vi "myRIO_BRig_FPGA_v3,81.vi"() -> ()   [LabVIEW 2014]
uses:
  <vilib>/rvi/Emulation/niFpgaGetClockAttributes.vi
  <vilib>/rvi/Emulation/niFpgaSctlEmulationGetInTimedLoop.vi
  <vilib>/rvi/Emulation/niFpgaEmulationReportErrorSimple.vi
  <vilib>/rvi/eio/common/nirviEmuTemplateMethod_errors.vi
  <vilib>/rvi/Emulation/niFpgaCriticalErrorInLSC.vi
  <vilib>/eio/EIONode/EIONode.xnode
panel:
  in  "L1Led_Baseline":bool
  in  "L2Led_Baseline":bool
  in  "CueLed_Baseline":bool
  in  "I_allReward":bool
  in  "AnaOut_1":u16
  in  "CueLed_Event":bool
  in  "CueLed_nValley":u32=100
  in  "CueLed_nPeak":u32=100
  in  "LC_Event_l2":bool
  in  "LC_Laser_l2":bool
  in  "LC_nShutter_l2":u32=100
  in  "LC_nValley_l2":u32=100
  in  "LC_nPeak_l2":u32=100
  in  "LR_wrong_nDelay_l2":u32
  in  "LR_reward_nDelay_l2":u32
  in  "LR_wrong_nTotal_l2":u32=100
  in  "LR_reward_nTotal_l2":u32=100
  in  "LR_wrong_laser_l2":bool
  in  "LR_wrong_Event_l2":bool
  in  "LR_reward_Laser_l2":bool
  in  "LR_reward_Event_l2":bool
  out "AnaIn_1":u16
  out "AnaIn_0":u16
  out "timeTrial_count":u32
  in  "timeTrial_trig":bool
  in  "k1__counter_per_ms":u16=100 min=100 max=40000 step=1
  in  "LC_nShutter_l1":u32=100
  in  "AnaOut_0":u16
  in  "LC_nValley_l1":u32=100
  in  "LC_nPeak_l1":u32=100
  in  "LC_Event_l1":bool
  in  "LR_wrong_nTotal_l1":u32=100
  in  "LR_wrong_nDelay_l1":u32
  in  "LR_reward_nTotal_l1":u32=100
  in  "LR_reward_nDelay_l1":u32
  in  "LR_reward_Event_l1":bool
  in  "LR_wrong_Event_l1":bool
  out "SelectWrong":bool
  out "SelectReward":bool
  in  "LR_wrong_Laser_l1":bool
  in  "LR_reward_Laser_l1":bool
  in  "Left(F)_or_Right(T)":bool
  in  "ignoreWrong":bool
  in  "SelectionState":bool
  in  "LC_Laser_l1":bool
  in  "FPGA_Stop":bool
  in  "audioTrigger_L":bool
  in  "audioTrigger_R":bool
  in  "audioFreq_L_kHz":u8=14 min=1 max=14 step=1
  in  "audioAmp_L":u16=1 min=1 max=32767 step=1
  in  "audioFreq_R_kHz":u8=14 min=1 max=14 step=1
  in  "audioAmp_R":u16=1 min=1 max=32767 step=1
  in  "A3_SL":bool
  in  "A1_SR":bool
  in  "Counts_Reset":bool
  out "A4_LickR":u32
  out "A2_LickL":u32
  in  "A6_Act":bool
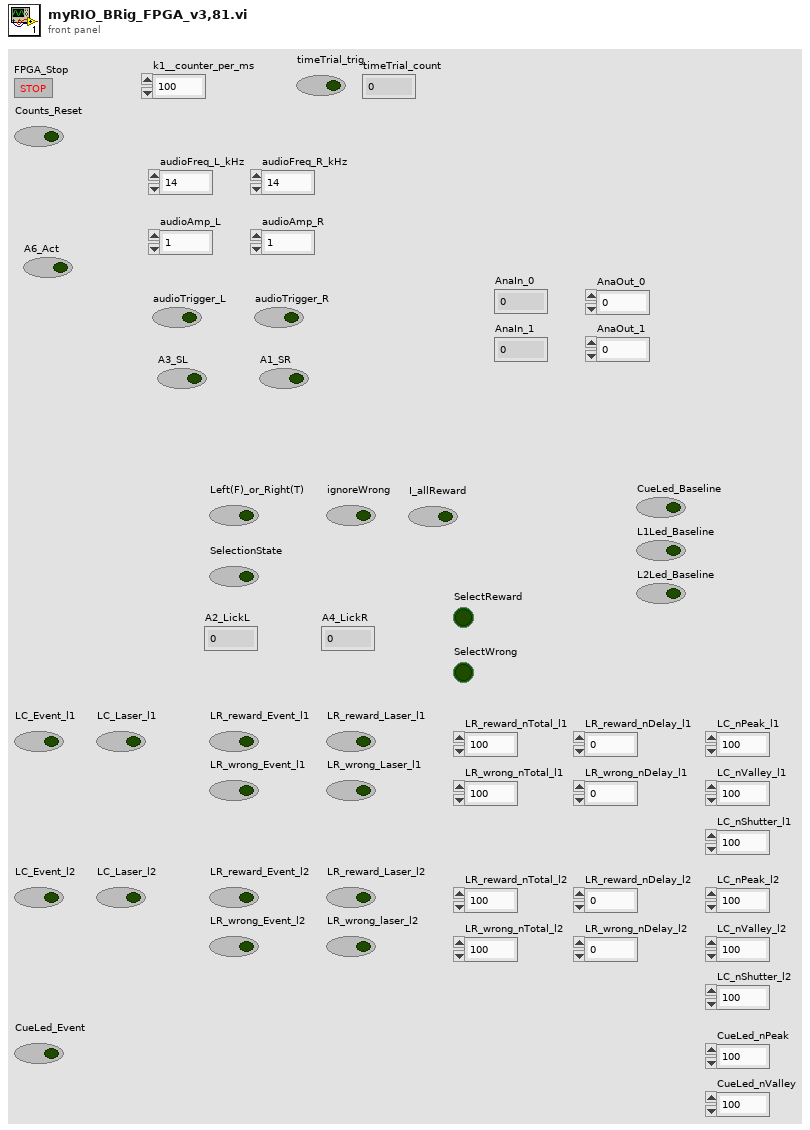
[diagram p1: front panel]
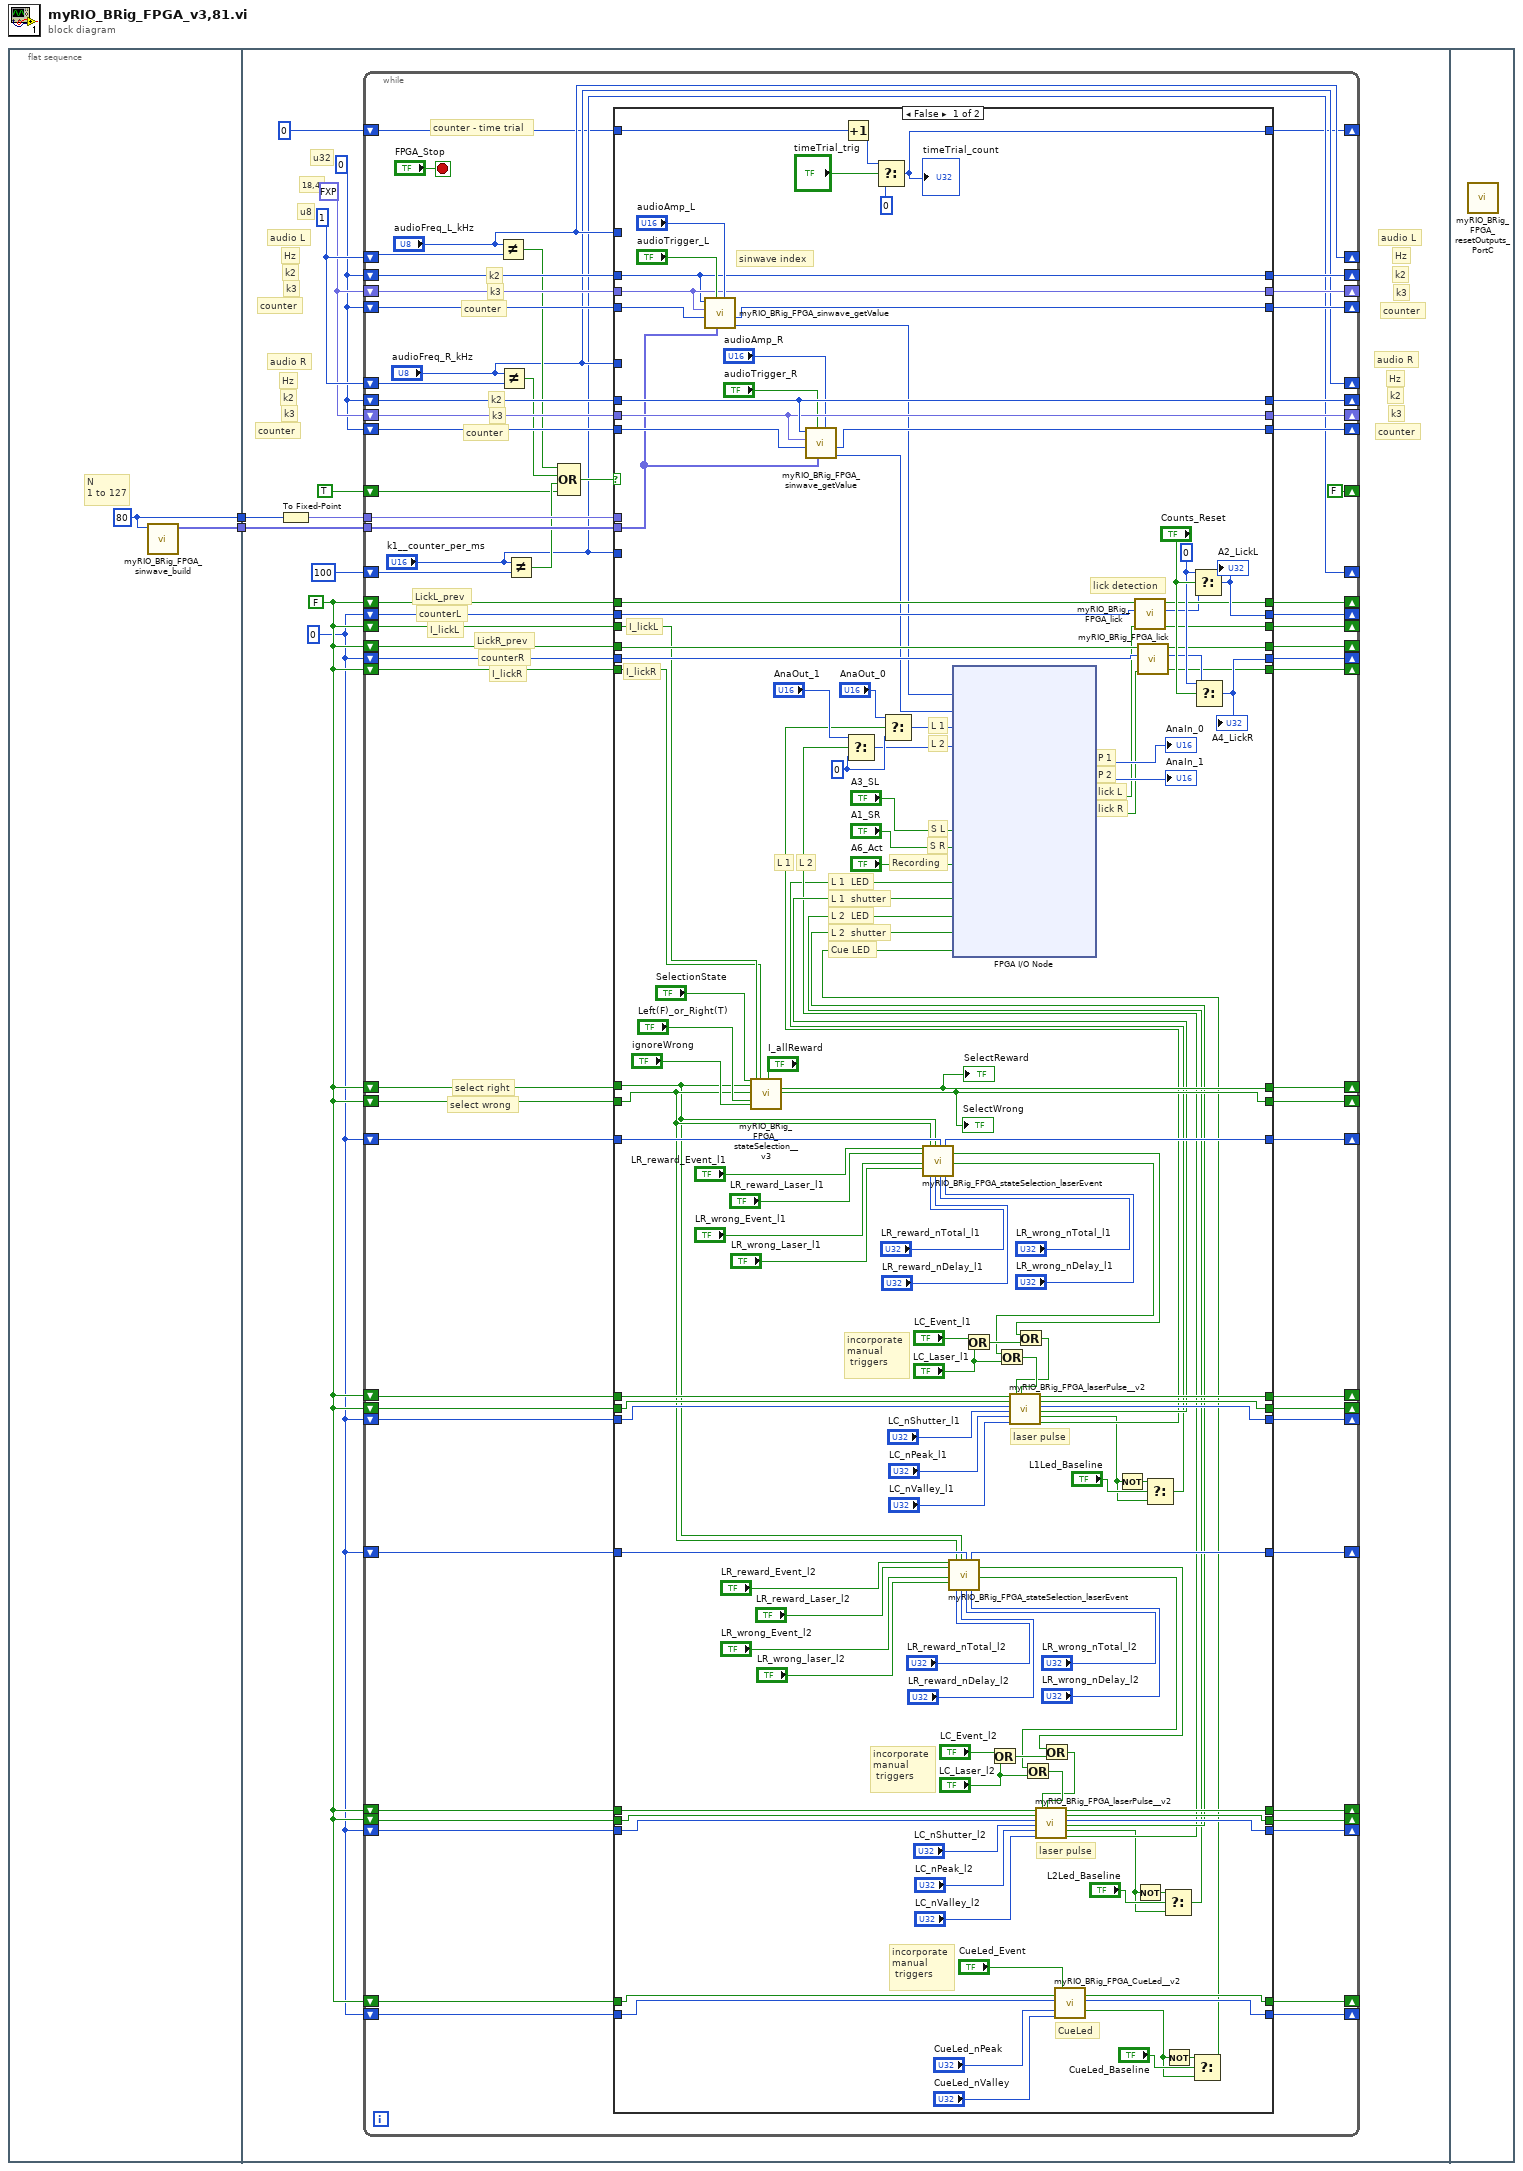
[diagram p0: block diagram]
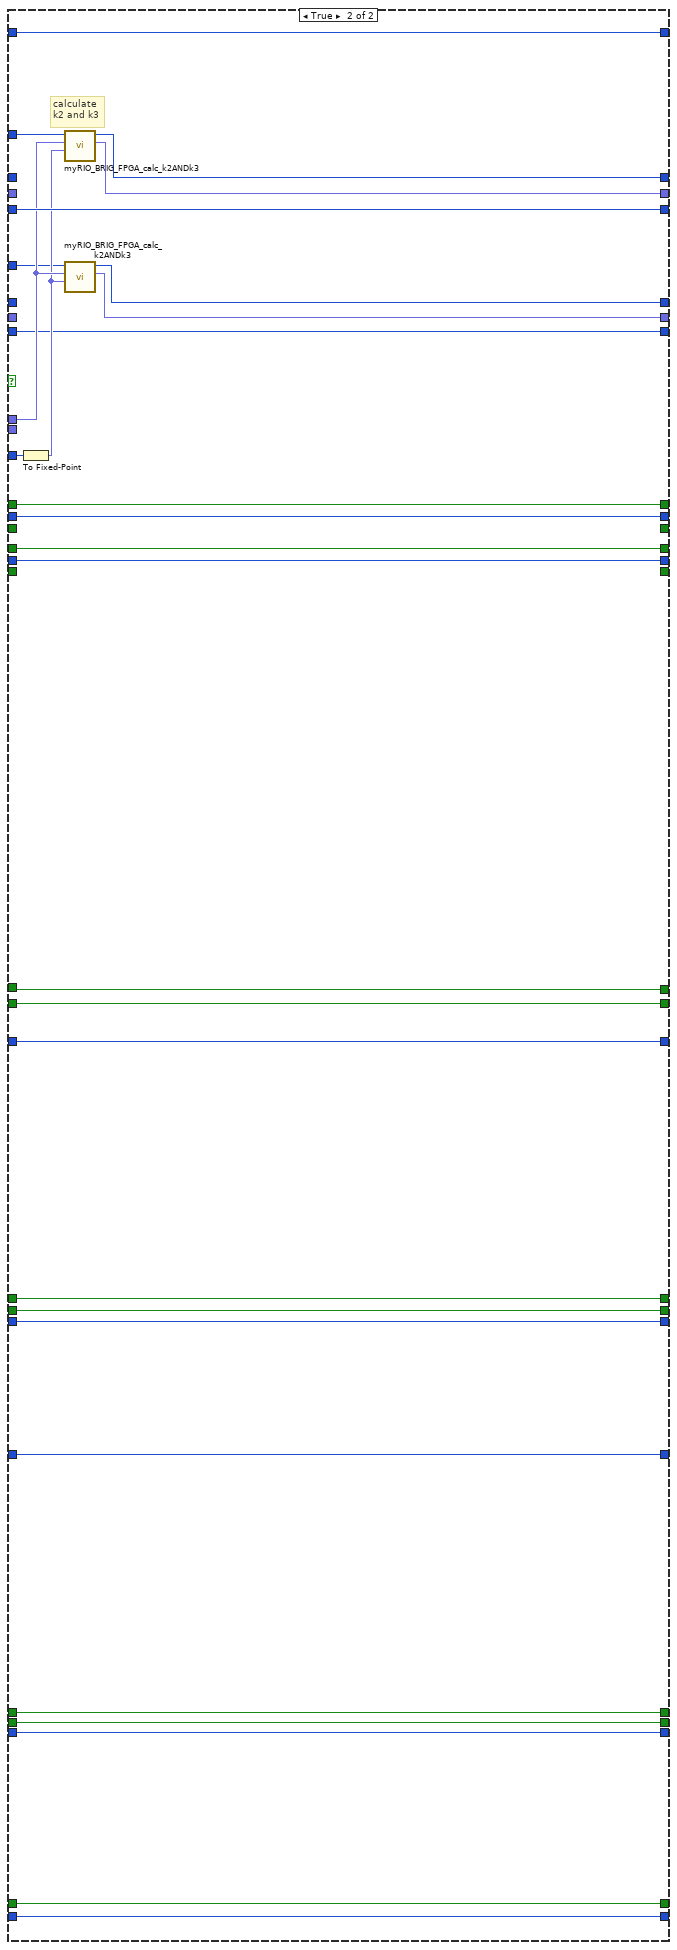
[diagram p2: hidden frame]
diagram:
  n1 = flat-sequence {
    tunnel: [w4] -> w2
    tunnel: [w3] -> w1
    tunnel: w2 -> [w15]
    tunnel: w1 -> [w14]
    frame #0 {
      w3 = 80 ("dimension size")
      # "N\n1 to 127"
      n2 = call "myRIO_BRig_FPGA_sinwave_build.vi"("input_Npts"=w3) -> ("output_array_sin"=w4:fxp<+/-,16,2>[])  [unwired: 10 in]
    }
    frame #1 {
      w5 = u32 0
      w6 = FALSE
      w10 = u32 0
      w11 = fxp<+,18,4> 0.0
      w12 = u8 1
      # "counter"
      # "k3"
      # "k2"
      # "counter"
      # "k3"
      # "k2"
      # "counter"
      # "counter"
      # "u32"
      # "k3"
      # "k2"
      # "k3"
      # "18,4"
      # "u8"
      # "Hz"
      # "Hz"
      # "audio R"
      # "audio L"
      # "Hz"
      # "k2"
      # "Hz"
      # "audio R"
      # "audio L"
      n3 = To Fixed-Point(number=w14) -> (fixed-point=w13:fxp<+,7,7>)  [unwired: 1 in]
      n4 = while {
        shift-right: ["audioFreq_L_kHz"] -> _
        shift-left: w12 -> [w80]
        shift-right: [w74] -> _
        shift-left: w10 -> [w78]
        shift-right: ["audioFreq_R_kHz"] -> _
        shift-left: w12 -> [w70]
        tunnel: w15 -> [w77]
        tunnel: w13 -> [w76]
        shift-right: [w73] -> _
        shift-left: w11 -> [w75]
        shift-right: [w71] -> _
        shift-left: w10 -> [w72]
        shift-right: [w68] -> _
        shift-left: w10 -> [w69]
        shift-right: [w66] -> _
        shift-left: w11 -> [w67]
        shift-right: [w64] -> _
        shift-left: w10 -> [w65]
        shift-right: ["k1__counter_per_ms"] -> _
        shift-left: u16 100 ("y") -> [w63]
        shift-right: [FALSE] -> _
        shift-left: TRUE -> [w58]
        shift-right: [w51] -> _
        shift-left: w6 -> [w53]
        shift-right: [w50] -> _
        shift-left: w6 -> [w52]
        shift-right: [w48] -> _
        shift-left: w5 -> [w49]
        shift-right: [w46] -> _
        shift-left: w5 -> [w47]
        shift-right: [w43] -> _
        shift-left: w6 -> [w45]
        shift-right: [w42] -> _
        shift-left: w6 -> [w44]
        shift-right: [w40] -> _
        shift-left: w6 -> [w41]
        shift-right: [w38] -> _
        shift-left: w6 -> [w39]
        shift-right: [w36] -> _
        shift-left: u32 0 -> [w37]
        shift-right: [w34] -> _
        shift-left: w5 -> [w35]
        shift-right: [w33] -> _
        shift-left: w6 -> [w30]
        shift-right: [w32] -> _
        shift-left: w6 -> [w29]
        shift-right: [w31] -> _
        shift-left: w5 -> [w28]
        shift-right: [w26] -> _
        shift-left: w5 -> [w27]
        shift-right: [w25] -> _
        shift-left: w6 -> [w22]
        shift-right: [w24] -> _
        shift-left: w6 -> [w21]
        shift-right: [w23] -> _
        shift-left: w5 -> [w20]
        shift-right: [w19] -> _
        shift-left: w6 -> [w17]
        shift-right: [w18] -> _
        shift-left: w5 -> [w16]
        stop <- "FPGA_Stop" stop-if-true
        # "counter"
        # "k3"
        # "k2"
        # "counter"
        # "k3"
        # "k2"
        # "counter - time trial"
        # "I_lickR"
        # "counterR"
        # "LickR_prev"
        # "I_lickL"
        # "counterL"
        # "LickL_prev"
        # "select wrong"
        # "select right"
        n5 = Not Equal?(x="audioFreq_L_kHz", y=w80) -> (x != y?=w62:bool)
        n6 = Not Equal?(x="audioFreq_R_kHz", y=w70) -> (x != y?=w61:bool)
        n7 = Not Equal?(x="k1__counter_per_ms", y=w63) -> (x != y?=w59:bool)
        n8 = Compound Arithmetic op=OR(w62, w61, w59, w58) -> (w60:bool)
        n9 = case shown="False" w60 {
          tunnel: w78 -> [w196 _]
          tunnel: "audioFreq_L_kHz" -> [_ w238]
          tunnel: w77 -> [w189 _]
          tunnel: w76 -> [_ w234]
          tunnel: "k1__counter_per_ms" -> [_ w239]
          tunnel: w75 -> [w197 _]
          tunnel: [w196 w237] -> w74
          tunnel: [w197 w236] -> w73
          tunnel: w72 -> [w201 w235]
          tunnel: [w198 w235] -> w71
          tunnel: w69 -> [w193 _]
          tunnel: [w193 w230] -> w68
          tunnel: w67 -> [w192 _]
          tunnel: [w192 w231] -> w66
          tunnel: w65 -> [w195 w229]
          tunnel: "audioFreq_R_kHz" -> [_ w232]
          tunnel: [w194 w229] -> w64
          tunnel: w53 -> [w184 w228]
          tunnel: w52 -> [w183 w227]
          tunnel: [w188 w228] -> w51
          tunnel: [w181 w227] -> w50
          tunnel: w49 -> [w185 w226]
          tunnel: [w211 w226] -> w48
          tunnel: w47 -> [w182 w225]
          tunnel: [w208 w225] -> w46
          tunnel: w45 -> [w123 w224]
          tunnel: w44 -> [w124 w223]
          tunnel: [w159 w224] -> w43
          tunnel: [w204 w223] -> w42
          tunnel: [w174 w220] -> w33
          tunnel: [w175 w219] -> w32
          tunnel: [w176 w218] -> w31
          tunnel: w41 -> [w178 _]
          tunnel: [w187 _] -> w40
          tunnel: w39 -> [w177 _]
          tunnel: [w179 _] -> w38
          tunnel: w37 -> [w166 w222]
          tunnel: [w163 w222] -> w36
          tunnel: w35 -> [w158 w221]
          tunnel: [w157 w221] -> w34
          tunnel: w30 -> [w148 w220]
          tunnel: w29 -> [w147 w219]
          tunnel: w28 -> [w146 w218]
          tunnel: w27 -> [w128 w217]
          tunnel: [w127 w217] -> w26
          tunnel: [w121 w216] -> w25
          tunnel: [w120 w215] -> w24
          tunnel: [w119 w214] -> w23
          tunnel: w22 -> [w118 w216]
          tunnel: w21 -> [w117 w215]
          tunnel: w20 -> [w116 w214]
          tunnel: [w113 w213] -> w19
          tunnel: [w112 w212] -> w18
          tunnel: w17 -> [w111 w213]
          tunnel: w16 -> [w110 w212]
          frame False {
            w108 = u16 0 ("f")
            w209 = u32 0 ("t")
            # "Cue LED"
            # "L 2  shutter"
            # "L 2  LED"
            # "L 2"
            # "L 1"
            # "L 1  shutter"
            # "L 1  LED"
            # "Recording"
            # "S L"
            # "S R"
            # "I_lickL"
            # "I_lickR"
            # "lick R"
            # "lick L"
            # "P 2"
            # "P 1"
            # "L 2"
            # "L 1"
            # "CueLed"
            # "incorporate\nmanual\n triggers"
            # "laser pulse"
            # "incorporate\nmanual\n triggers"
            # "sinwave index"
            # "lick detection"
            # "laser pulse"
            # "incorporate\nmanual\n triggers"
            n10 = call "myRIO_BRig_FPGA_sinwave_getValue.vi"("audioAmp"="audioAmp_L", "sinwave"=w189, "audioTrigger"="audioTrigger_L", "counter"=w201, "k3"=w197, "k2"=w196) -> ("output_audioValue"=w161:i16, "output_counter"=w198:u32)  [unwired: 4 in]
            n11 = call "myRIO_BRig_FPGA_stateSelection__v3.vi"("I_selectionState"="SelectionState", "I_selectRight"=w123, "I_selectWrong"=w124, "I_Left(F)_or_Right(T)"="Left(F)_or_Right(T)", "I_ignoreWrong"="ignoreWrong", "I_lickL"=w178, "I_lickR"=w177, "I_allReward"="I_allReward") -> ("output__I_selectRight"=w159:bool, "output__I_selectWrong"=w204:bool)  [unwired: 18 in]
            "SelectWrong" <- w204
            "SelectReward" <- w159
            n12 = call "myRIO_BRig_FPGA_sinwave_getValue.vi"("audioAmp"="audioAmp_R", "sinwave"=w189, "audioTrigger"="audioTrigger_R", "counter"=w195, "k3"=w192, "k2"=w193) -> ("output_audioValue"=w160:i16, "output_counter"=w194:u32)  [unwired: 4 in]
            n13 = Increment(x=w166) -> (x+1=w165:u32)
            n14 = Select(t=w165, s="timeTrial_trig", f=u32 0) -> (s? t:f=w163:u32)
            "timeTrial_count" <- w163
            n15 = call "myRIO_BRig_FPGA_stateSelection_laserEvent.vi"("I_LR_reward"="LR_reward_Event_l1", "I_LR_reward_laser"="LR_reward_Laser_l1", "I_LR_wrong"="LR_wrong_Event_l1", "I_LR_wrong_laser"="LR_wrong_Laser_l1", "I_selectWrong"=w124, "laser_reward_nTotal"="LR_reward_nTotal_l1", "I_selectReward"=w123, "laser_reward_nDelay"="LR_reward_nDelay_l1", "counter"=w158, "laser_wrong_nTotal"="LR_wrong_nTotal_l1", "laser_wrong_nDelay"="LR_wrong_nDelay_l1") -> ("output_counter"=w157:u32, "output_I_laserEvent"=w145:bool, "output_I_laserOn"=w144:bool)  [unwired: 6 in]
            n16 = call "myRIO_BRig_FPGA_stateSelection_laserEvent.vi"("I_LR_reward"="LR_reward_Event_l2", "I_LR_reward_laser"="LR_reward_Laser_l2", "I_LR_wrong"="LR_wrong_Event_l2", "I_LR_wrong_laser"="LR_wrong_laser_l2", "I_selectWrong"=w124, "laser_reward_nTotal"="LR_reward_nTotal_l2", "I_selectReward"=w123, "laser_reward_nDelay"="LR_reward_nDelay_l2", "counter"=w128, "laser_wrong_nTotal"="LR_wrong_nTotal_l2", "laser_wrong_nDelay"="LR_wrong_nDelay_l2") -> ("output_counter"=w127:u32, "output_I_laserEvent"=w122:bool, "output_I_laserOn"=w129:bool)  [unwired: 6 in]
            n17 = Or(x="LC_Event_l1", y="LC_Laser_l1") -> (x .or. y?=w170:bool)
            n18 = Or(x="LC_Event_l2", y="LC_Laser_l2") -> (x .or. y?=w139:bool)
            n19 = Or(x=w144, y="LC_Laser_l1") -> (x .or. y?=w168:bool)
            n20 = Or(x=w145, y=w170) -> (x .or. y?=w167:bool)
            n21 = call "myRIO_BRig_FPGA_laserPulse__v2.vi"("I_shutter"=w148, "I_peak"=w147, "count"=w146, "laser_Nshutter"="LC_nShutter_l1", "laser_Npeak"="LC_nPeak_l1", "laser_Nvalley"="LC_nValley_l1", "I_laserEvent"=w167, "I_laser"=w168) -> ("output_I_shutter"=w174:bool, "output_I_peak"=w175:bool, "output_count"=w176:u32, "output_shutter"=w94:bool, "output_led"=w84:bool, "output_laser"=w93:bool)  [unwired: 6 in]
            n22 = Select(t="AnaOut_0", s=w93, f=w108) -> (s? t:f=w103:u16)
            n23 = Or(x=w129, y="LC_Laser_l2") -> (x .or. y?=w137:bool)
            n24 = Or(x=w122, y=w139) -> (x .or. y?=w136:bool)
            n25 = call "myRIO_BRig_FPGA_laserPulse__v2.vi"("I_shutter"=w118, "I_peak"=w117, "count"=w116, "laser_Nshutter"="LC_nShutter_l2", "laser_Npeak"="LC_nPeak_l2", "laser_Nvalley"="LC_nValley_l2", "I_laserEvent"=w136, "I_laser"=w137) -> ("output_I_shutter"=w121:bool, "output_I_peak"=w120:bool, "output_count"=w119:u32, "output_shutter"=w92:bool, "output_led"=w88:bool, "output_laser"=w91:bool)  [unwired: 6 in]
            n26 = Select(t="AnaOut_1", s=w91, f=w108) -> (s? t:f=w102:u16)
            n27 = call "myRIO_BRig_FPGA_CueLed__v2.vi"("I_peak"=w111, "count"=w110, "laser_Npeak"="CueLed_nPeak", "laser_Nvalley"="CueLed_nValley", "I_CueLed_Event"="CueLed_Event") -> ("output_I_peak"=w113:bool, "output_count"=w112:u32, "output_led"=w82:bool)  [unwired: 12 in]
            n28 = Not(x=w84) -> (.not. x?=w86:bool)
            n29 = Not(x=w88) -> (.not. x?=w90:bool)
            n30 = Select(t=w86, s="L1Led_Baseline", f=w84) -> (s? t:f=w83:bool)
            n31 = Select(t=w90, s="L2Led_Baseline", f=w88) -> (s? t:f=w87:bool)
            n32 = Not(x=w82) -> (.not. x?=w105:bool)
            n33 = Select(t=w105, s="CueLed_Baseline", f=w82) -> (s? t:f=w81:bool)
            n34 = xnode "FPGA I/O Node"("AudioOut/Left"=w161, "AudioOut/Right"=w160, "ConnectorB/AO0"=w103, "ConnectorB/AO1"=w102, "ConnectorA/DIO3"="A3_SL", "ConnectorA/DIO5"="A1_SR", "ConnectorA/DIO0"="A6_Act", "ConnectorB/DIO14"=w83, "ConnectorA/DIO6"=w94, "ConnectorB/DIO15"=w87, "ConnectorA/DIO7"=w92, "ConnectorA/DIO9"=w81) -> ("ConnectorB/AI1"=→"AnaIn_0":u16, "ConnectorB/AI2"=→"AnaIn_1":u16, "ConnectorA/DIO4"=w99:bool, "ConnectorA/DIO2"=w98:bool)  [unwired: 16 in, 16 out]
            n35 = call "myRIO_BRig_FPGA_lick.vi"("I_stateDetector_new"=w99, "counter"=w185, "I_stateDetector_prev"=w184) -> ("output_I_lick"=w187:bool, "output_counter"=w186:u32, "output_I_stateDetector_prev"=w188:bool)  [unwired: 6 in]
            n36 = call "myRIO_BRig_FPGA_lick.vi"("I_stateDetector_new"=w98, "counter"=w182, "I_stateDetector_prev"=w183) -> ("output_I_lick"=w179:bool, "output_counter"=w180:u32, "output_I_stateDetector_prev"=w181:bool)  [unwired: 6 in]
            n37 = Select(t=w209, s="Counts_Reset", f=w186) -> (s? t:f=w211:u32)
            "A2_LickL" <- w211
            n38 = Select(t=w209, s="Counts_Reset", f=w180) -> (s? t:f=w208:u32)
            "A4_LickR" <- w208
          }
          frame True {
            # "calculate\nk2 and k3"
            n39 = To Fixed-Point(number=w239) -> (fixed-point=w233:fxp<+,16,16>)  [unwired: 1 in]
            n40 = call "myRIO_BRIG_FPGA_calc_k2ANDk3.vi"("input_k1[count/ms]"=w233, "input_Npts"=w234, "input_freq[kHz]"=w238) -> ("output_k3"=w236:fxp<+,18,4>, "output_k2"=w237:u32)  [unwired: 7 in]
            n41 = call "myRIO_BRIG_FPGA_calc_k2ANDk3.vi"("input_k1[count/ms]"=w233, "input_Npts"=w234, "input_freq[kHz]"=w232) -> ("output_k3"=w231:fxp<+,18,4>, "output_k2"=w230:u32)  [unwired: 7 in]
          }
        }
      }
    }
    frame #2 {
      n42 = call "myRIO_BRig_FPGA_resetOutputs_PortC.vi"() -> ()  [unwired: 12 in]
    }
  }
